vi "GOOP_ApplyOverlayIconFromClassRef.vi"(8 "error in (no error)":errorcluster, 11 "LVClassRef":refnum<vi>) -> (0 "error out":errorcluster)   [LabVIEW 2020]
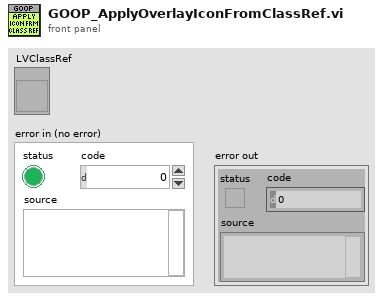
[diagram p1: front panel]
types:
  T1 = cluster{"Item URL":string, "Item ID":string, "Item Index":i32, "Specific Type":string}
  T2 = typedef "ItemRef.ctl" = u64
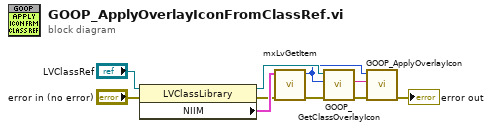
[diagram p0: block diagram]
diagram:
  n1 = property class="LVClassLibrary"(reference="LVClassRef", error in="error in (no error)") -> (reference out=w8:refnum<vi>, error out=w4:errorcluster, "NIIM"=w9:T1)
  n2 = call <resource>:"mxLvGetItem.vi"("error in"=w4, "NIIM"=w9) -> ("error out"=w5:errorcluster, "Item"=w3:T2)  [unwired: 8 in]
  n3 = call "GOOP_GetClassOverlayIcon.vi"("error in (no error)"=w5, "Item"=w3, "LVClassLibrary in"=w8) -> ("error out"=w7:errorcluster, "IconName"=w6:string)  [unwired: 6 in, 1 out]
  n4 = call "GOOP_ApplyOverlayIcon.vi"("error in (no error)"=w7, "IconName(NoPngExtension)"=w6, "Object"=w3) -> ("error out"=→"error out":errorcluster)  [unwired: 8 in]
